vi "PathPlanner_RotationTarget_FromJSON.vi"(11 "JSON Object":string) -> (3 "RotationTarget":T1={"target"={"VALUE"=0.0, "COS"=1.0, "SIN"=0.0}, "WaypointRelativePosition"=0.0, "Exists"=FALSE} {"target"."SIN" format="%13.4f"; "target"."COS" format="%13.4f"; "target"."VALUE" format="%13.4f"})   [LabVIEW 2019, in "PathPlanner24.lvlib"]
doc: "/**\n * Create a path constraints object from json\n *\n * @param constraintsJson {@link org.json.simple.JSONObject} representing a path constraints\n * object\n * @return The path constraints defined by the given json\n */"
uses:
  PathPlanner24.lvlib
  TypeDef/PathPlannerRotationTarget.ctl
  <vilib>/Rock Robotics/WPI/ThirdParty/JAS_Junk/TrajLib/TypeDef/ROTATION2D.ctl
  <vilib>/Rock Robotics/WPI/ThirdParty/JAS_Junk/TrajLib/Trajectory_Library.lvlib
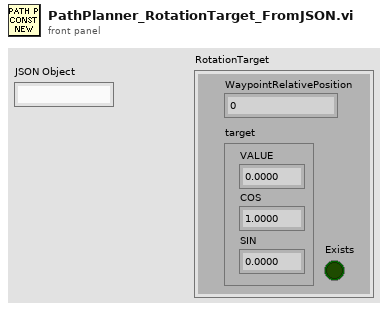
[diagram p1: front panel]
types:
  T1 = typedef "PathPlanner24.lvlib/PathPlannerRotationTarget.ctl" = cluster{"target":T2, "WaypointRelativePosition":dbl, "Exists":bool}
  T2 = typedef "Trajectory_Library.lvlib/ROTATION2D.ctl" = cluster{"VALUE":dbl, "COS":dbl, "SIN":dbl}
  T3 = cluster{"target":T2, "WaypointRelativePosition":dbl}
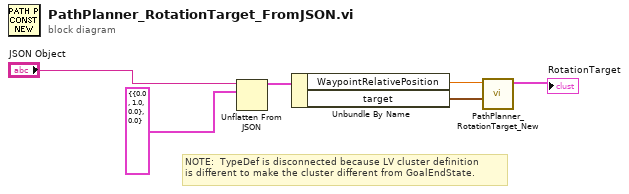
[diagram p0: block diagram]
diagram:
  # "NOTE:  TypeDef is disconnected because LV cluster definition\nis different to make the cluster different from GoalEndState."
  n1 = Unflatten From JSON(JSON string="JSON Object", type and defaults=T3 {"target"={"VALUE"=0.0, "COS"=1.0, "SIN"=0.0}, "WaypointRelativePosition"=0.0} ("RotationTarget")) -> (value=w4:T3)  [unwired: 5 in, 1 out]
  n2 = Unbundle By Name(w4) -> ("WaypointRelativePosition"=w3:dbl, "target"=w2:T2)
  n3 = call "PathPlanner_RotationTarget_New.vi"("target"=w2, "WaypointRelativePosition"=w3) -> ("RotationTarget"=→"RotationTarget":T1)  [unwired: 9 in]
